vi "Build DashBoard Data.vi"(11 "Dashboard Enables":T2={"TargetInView"=TRUE, "AlignedToTarget"=FALSE, "TopBall"=TRUE, "MidBall"=FALSE, "BotBall"=TRUE, "OKToShoot"=FALSE, "DistanceToTarget"=FALSE, "AngleOfConveyor"=FALSE}) -> ()   [LabVIEW 2011]
doc: "This VI builds data and sends it back to the dashboard PC program. By default it sends back the raw values for the first analog, digital, and solenoid module. Modify it to send back the data you want to view. Consider adding higher level data to the Dashboard Datatype.ctl and to this VI. Then update the Dashboard to display the data however you like.\n\nThis software is licensed. Open the labview\\readme\\WPI Robotics Library Open Source License.txt file for more information."
uses:
  DashboardEnable.ctl
  Dashboard Datatype.ctl
  Robot Global Data.vi
panel:
  out "Dashboard Data":T1
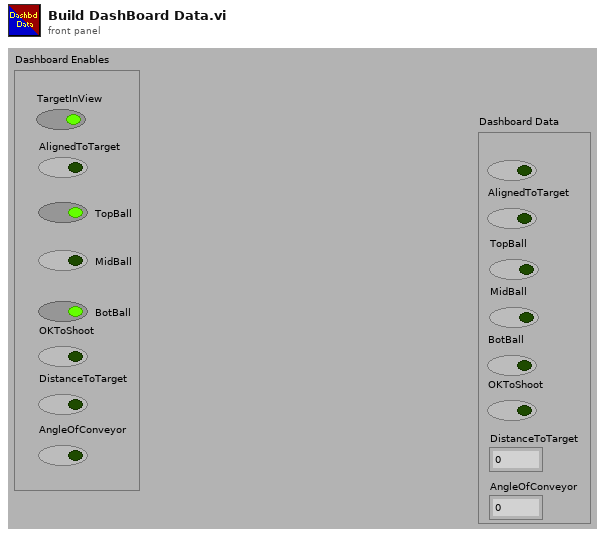
[diagram p1: front panel]
types:
  T1 = typedef "Dashboard Datatype.ctl" = cluster{"TargetInView":bool, "AlignedToTarget":bool, "TopBall":bool, "MidBall":bool, "BotBall":bool, "OKToShoot":bool, "DistanceToTarget":dbl, "AngleOfConveyor":dbl}
  T2 = typedef "DashboardEnable.ctl" = cluster{"TargetInView":bool, "AlignedToTarget":bool, "TopBall":bool, "MidBall":bool, "BotBall":bool, "OKToShoot":bool, "DistanceToTarget":bool, "AngleOfConveyor":bool}
  T3 = cluster{"Position":cluster{"X":dbl, "Y":dbl}, "Distance (ft)":dbl}
  T4 = typedef "WPI_DigitalInputDevRef.ctl" = cluster{"DevStatus":errorcluster, "DIO Channel":T5, "Digital Module":T6}
  T5 = typedef "FPGA_DIOChannel.ctl" = enum8{"DIO 1", "DIO 2", "DIO 3", "DIO 4", "DIO 5", "DIO 6", "DIO 7", "DIO 8", "DIO 9", "DIO 10", "DIO 11", "DIO 12", "DIO 13", "DIO 14", "Invalid"}
  T6 = typedef "FPGA_TypedefDigitalModule.ctl" = enum16{"Digital Module 1", "Digital Module 2"}
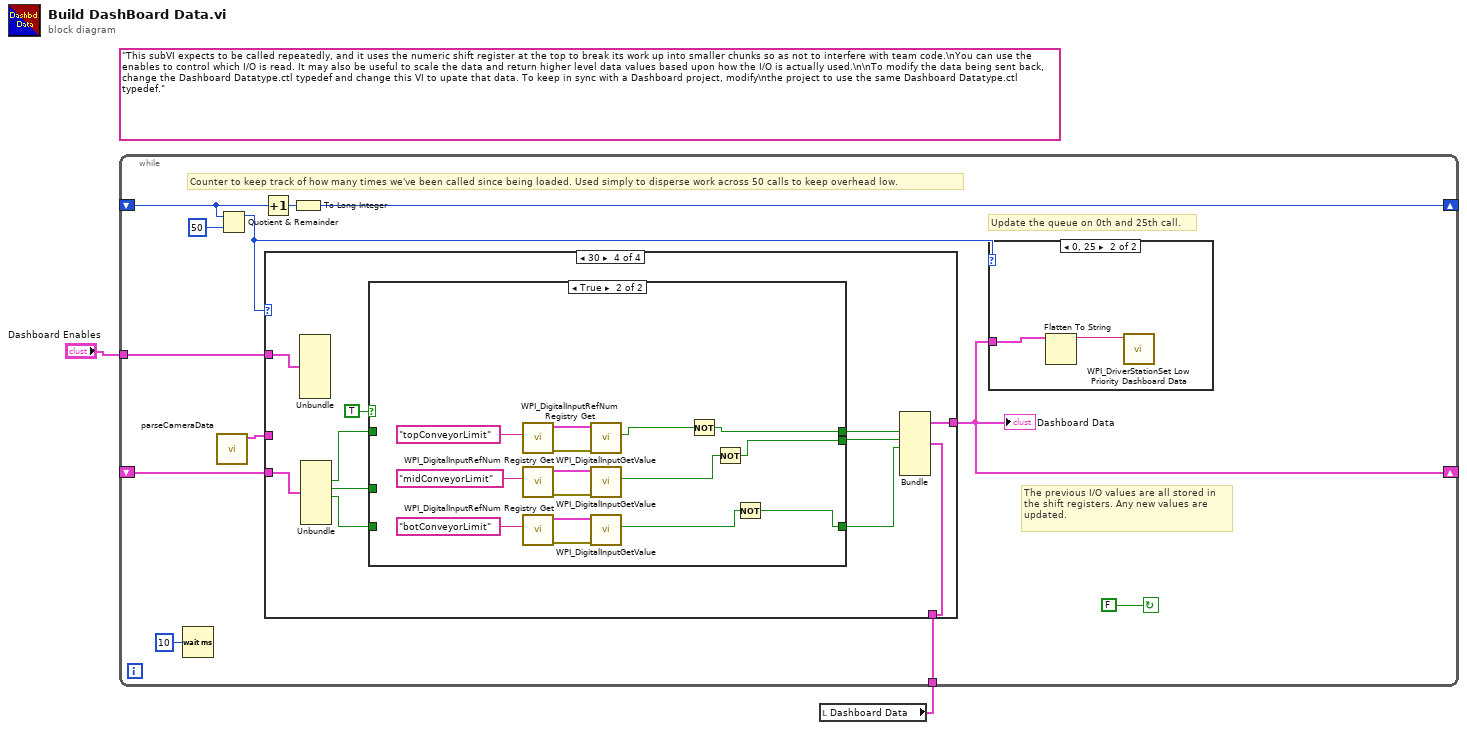
[diagram p0: block diagram]
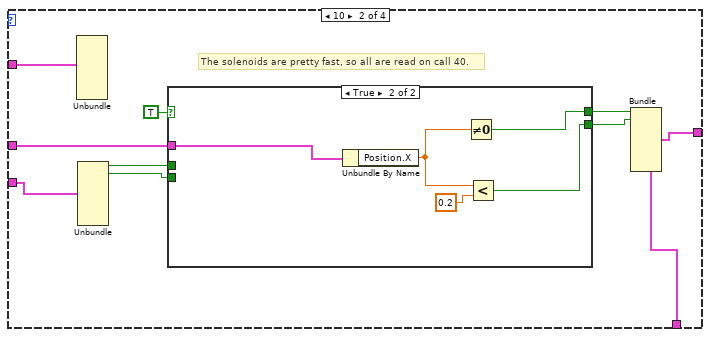
[diagram p4: hidden frame]
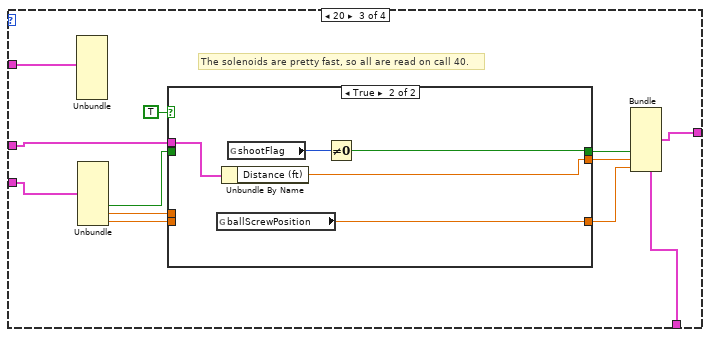
[diagram p6: hidden frame]
diagram:
  (unwired) "This subVI expects to be called repeatedly, and it uses the numeric shift register at the top to break its work up into smaller chunks so as not to interfere with team code.\nYou can use the enables to control which I/O is read. It may also be useful to scale the data and return higher level data values based upon how the I/O is actually used.\n\nTo modify the data being sent back, change the Dashboard Datatype.ctl typedef and change this VI to upate that data. To keep in sync with a Dashboard project, modify\nthe project to use the same Dashboard Datatype.ctl typedef."
  n1 = local read "Dashboard Data"() -> (w1:T1)
  n2 = while {
    shift-right: [w8] -> _
    shift-left: _ -> [w10]
    shift-right: [w5] -> _
    shift-left: _ -> [w12]
    tunnel: w1 -> [w7]
    tunnel: "Dashboard Enables" -> [w6]
    stop <- FALSE continue-if-true
    # "Counter to keep track of how many times we've been called since being loaded. Used simply to disperse work across 50 calls to keep overhead low."
    # "Update the queue on 0th and 25th call."
    # "The previous I/O values are all stored in\nthe shift registers. Any new values are\nupdated."
    n3 = Wait (ms)(milliseconds to wait=u32 10) -> ()  [unwired: 1 out]
    n4 = call "parseCameraData.vi"() -> ("TargetInfoOut"=w4:T3)  [unwired: 11 in]
    n5 = Quotient & Remainder(x=w10, y=50) -> (x-y*floor(x/y)=w9:i32)  [unwired: 1 out]
    n6 = Increment(x=w10) -> (x+1=w14:i32)
    n7 = case shown="30" w9 {
      tunnel: [w17 w27 w46 w63] -> w5
      tunnel: w12 -> [w17 w24 w43 w64]
      tunnel: w7 -> [_ w26 w45 w62]
      tunnel: w6 -> [_ w25 w44 w65]
      tunnel: w4 -> [_ w19 w36 _]
      frame Default {
        # "Don't update any I/O"
      }
      frame 10 {
        # "The solenoids are pretty fast, so all are read on call 40."
        n8 = Unbundle(w25) -> ()  [unwired: 8 out]
        n9 = Unbundle(w24) -> ("TargetInView"=w21:bool, "AlignedToTarget"=w20:bool)  [unwired: 6 out]
        n10 = case shown="True" TRUE {
          tunnel: [w29 w34] -> w23
          tunnel: [w28 w31] -> w22
          tunnel: w21 -> [w29 _]
          tunnel: w20 -> [w28 _]
          tunnel: w19 -> [_ w30]
          frame False {
          }
          frame True {
            n11 = Unbundle By Name(w30) -> ("Position.X"=w33:dbl)
            n12 = Not Equal To 0?(x=w33) -> (x != 0?=w34:bool)
            n13 = Less?(x=w33, y=0.2) -> (x < y?=w31:bool)
          }
        }
        n14 = Bundle(cluster=w26, "TargetInView"=w23, "AlignedToTarget"=w22) -> (w27:T1)  [unwired: 6 out]
      }
      frame 20 {
        # "The solenoids are pretty fast, so all are read on call 40."
        n15 = Unbundle(w44) -> ()  [unwired: 8 out]
        n16 = Unbundle(w43) -> ("OKToShoot"=w42:bool, "DistanceToTarget"=w40:dbl, "AngleOfConveyor"=w37:dbl)  [unwired: 5 out]
        n17 = case shown="True" TRUE {
          tunnel: w42 -> [w49 _]
          tunnel: [w49 w53] -> w39
          tunnel: [w48 w51] -> w41
          tunnel: w40 -> [w48 _]
          tunnel: [w47 w50] -> w38
          tunnel: w37 -> [w47 _]
          tunnel: w36 -> [_ w52]
          frame False {
          }
          frame True {
            n18 = global read "Robot Global Data.vi" "ballScrewPosition"() -> (w50:dbl)
            n19 = Unbundle By Name(w52) -> ("Distance (ft)"=w51:dbl)
            n20 = global read "Robot Global Data.vi" "shootFlag"() -> (w54:u8)
            n21 = Not Equal To 0?(x=w54) -> (x != 0?=w53:bool)
          }
        }
        n22 = Bundle(cluster=w45, "OKToShoot"=w39, "DistanceToTarget"=w41, "AngleOfConveyor"=w38) -> (w46:T1)  [unwired: 5 out]
      }
      frame 30 {
        n23 = Unbundle(w65) -> ()  [unwired: 8 out]
        n24 = Unbundle(w64) -> ("TopBall"=w58:bool, "MidBall"=w57:bool, "BotBall"=w56:bool)  [unwired: 5 out]
        n25 = case shown="True" TRUE {
          tunnel: [w68 w69] -> w61
          tunnel: [w67 w71] -> w60
          tunnel: [w66 w73] -> w59
          tunnel: w58 -> [w68 _]
          tunnel: w57 -> [w67 _]
          tunnel: w56 -> [w66 _]
          frame False {
          }
          frame True {
            n26 = call <vilib>:"WPI_DigitalInputRefNum Registry Get.vi"("refnum name"="topConveyorLimit") -> ("error out"=w80:errorcluster, "DigitalInputDevRef"=w79:T4)  [unwired: 9 in]
            n27 = call <vilib>:"WPI_DigitalInputRefNum Registry Get.vi"("refnum name"="midConveyorLimit") -> ("error out"=w76:errorcluster, "DigitalInputDevRef"=w75:T4)  [unwired: 9 in]
            n28 = call <vilib>:"WPI_DigitalInputRefNum Registry Get.vi"("refnum name"="botConveyorLimit") -> ("error out"=w77:errorcluster, "DigitalInputDevRef"=w78:T4)  [unwired: 9 in]
            n29 = call <vilib>:"WPI_DigitalInputGetValue.vi"("error in (no error)"=w80, "DigitalInputDevRef"=w79) -> ("Value"=w70:bool)  [unwired: 7 in, 2 out]
            n30 = call <vilib>:"WPI_DigitalInputGetValue.vi"("error in (no error)"=w76, "DigitalInputDevRef"=w75) -> ("Value"=w72:bool)  [unwired: 7 in, 2 out]
            n31 = call <vilib>:"WPI_DigitalInputGetValue.vi"("error in (no error)"=w77, "DigitalInputDevRef"=w78) -> ("Value"=w74:bool)  [unwired: 7 in, 2 out]
            n32 = Not(x=w70) -> (.not. x?=w69:bool)
            n33 = Not(x=w72) -> (.not. x?=w71:bool)
            n34 = Not(x=w74) -> (.not. x?=w73:bool)
          }
        }
        n35 = Bundle(cluster=w62, "TopBall"=w61, "MidBall"=w60, "BotBall"=w59) -> (w63:T1)  [unwired: 5 out]
      }
    }
    "Dashboard Data" <- w5
    n36 = To Long Integer(number=w14) -> (32bit integer=w8:i32)
    n37 = case shown="0, 25" w9 {
      tunnel: w5 -> [_ w16]
      frame Default {
      }
      frame 0, 25 {
        n38 = Flatten To String(anything=w16) -> (data string=w15:string)  [unwired: 1 in, 4 out]
        n39 = call <vilib>:"WPI_DriverStationSet Low Priority Dashboard Data.vi"("User Data"=w15) -> ()  [unwired: 1 in, 10 out]
      }
    }
  }
